vi "SO55 Settings.vi"(0 "Error In":errorcluster) -> (1 "Settings Out":T1, 2 "Error Out":errorcluster)   [LabVIEW 2012]
panel:
  in  "OK Button":bool
  in  "Settings In":T1
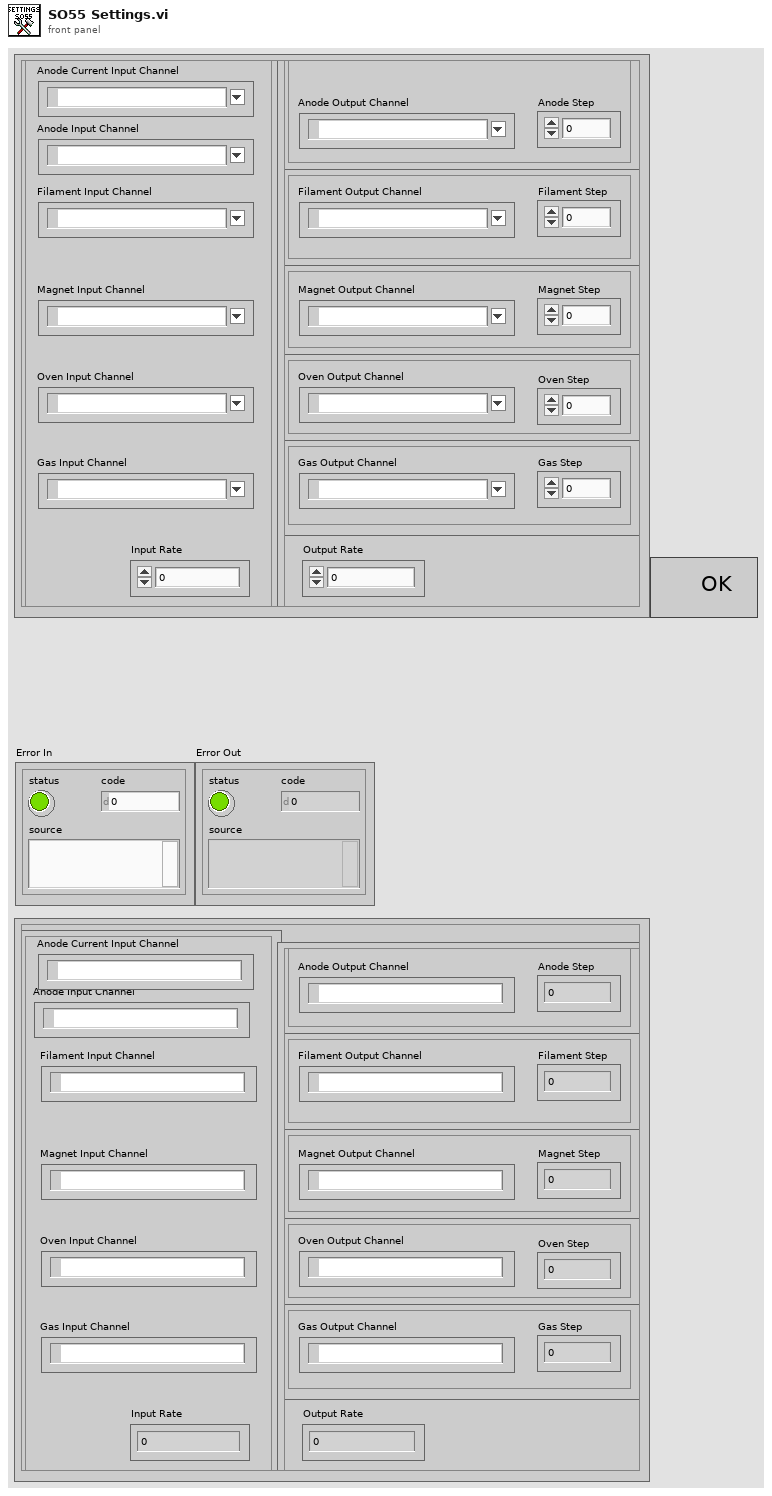
[diagram p1: front panel]
types:
  T1 = cluster{"Input":cluster{"Anode Input Channel":tag, "Filament Input Channel":tag, "Magnet Input Channel":tag, "Oven Input Channel":tag, "Gas Input Channel":tag, "Input Rate":dbl, "Anode Current Input Channel":tag}, "Output":cluster{"Anode":cluster{"Anode Output Channel":tag, "Anode Step":dbl}, "Filament":cluster{"Filament Output Channel":tag, "Filament Step":dbl}, "Magnet":cluster{"Magnet Output Channel":tag, "Magnet Step":dbl}, "Oven":cluster{"Oven Output Channel":tag, "Oven Step":dbl}, "Gas":cluster{"Gas Output Channel":tag, "Gas Step":dbl}, "Output Rate":dbl}}
  T2 = enum16{"open", "replace", "create", "open or create", "replace or create", "replace or create with confirmation"}
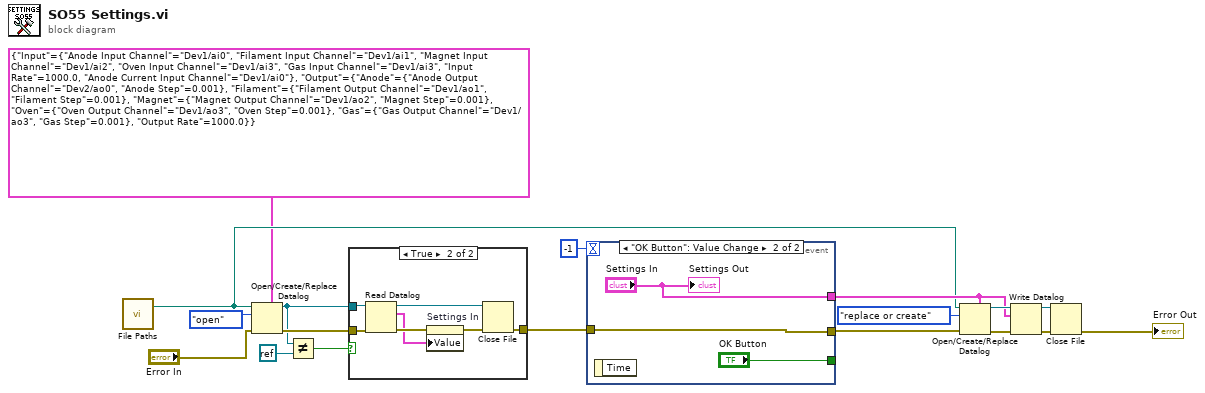
[diagram p0: block diagram]
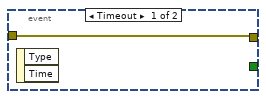
[diagram p2: hidden frame]
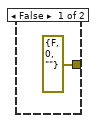
[diagram p3: hidden frame]
diagram:
  n1 = call "File Paths.vi"() -> ("SO55 Settings path"=w3:path)  [unwired: 1 out]
  n2 = Open/Create/Replace Datalog(5:T1 {"Input"={"Anode Input Channel"="Dev1/ai0", "Filament Input Channel"="Dev1/ai1", "Magnet Input Channel"="Dev1/ai2", "Oven Input Channel"="Dev1/ai3", "Gas Input Channel"="Dev1/ai3", "Input Rate"=1000.0, "Anode Current Input Channel"="Dev1/ai0"}, "Output"={"Anode"={"Anode Output Channel"="Dev2/ao0", "Anode Step"=0.001}, "Filament"={"Filament Output Channel"="Dev1/ao1", "Filament Step"=0.001}, "Magnet"={"Magnet Output Channel"="Dev1/ao2", "Magnet Step"=0.001}, "Oven"={"Oven Output Channel"="Dev1/ao3", "Oven Step"=0.001}, "Gas"={"Gas Output Channel"="Dev1/ao3", "Gas Step"=0.001}, "Output Rate"=1000.0}}, 8:"Error In", 10:T2."open" ("operation (0:open)"), 11:w3) -> (0:w16:errorcluster, 3:w15:refnum<k1>)  [unwired: 2 in, 1 out]
  n3 = Not Equal?(x=w15, y=refnum<k0> refnum) -> (x != y?=w17:bool)
  n4 = case shown="True" w17 {
    tunnel: w16 -> [_ w26]
    tunnel: w15 -> [_ w21]
    tunnel: [errorcluster {"status"=FALSE, "code"=0, "source"=""} ("error out") w22] -> w13
    frame False {
    }
    frame True {
      n5 = Read Datalog(4:w26, 7:w21) -> (0:w25:errorcluster, 2:w20:T1, 3:w23:refnum<k1>)  [unwired: 1 in]
      n6 = property on="Settings In" class="Clust (strict)"(error in=w25, "Value"=w20) -> (error out=w24:errorcluster)  [unwired: 1 in, 1 out]
      n7 = Close File(refnum=w23, error in=w24) -> (error out=w22:errorcluster)  [unwired: 1 out]
    }
  }
  n8 = event shown="[1] \"OK Button\": Value Change" {
    selector: _ -> [_ _]
    dyn-events: _ -> [_ _]
    timeout: -1 -> [_ _]
    tunnel: w13 -> [w27 w29]
    tunnel: [_ "OK Button"] -> _
    tunnel: [w27 w29] -> w11
    tunnel: [_ "Settings In"] -> w5
    event Timeout {
      n9 = event-data() -> ()  [unwired: 1 in, 2 out]
    }
    event "OK Button": Value Change {
      n10 = event-data() -> ()  [unwired: 1 in, 1 out]
      "Settings Out" <- "Settings In"
    }
  }
  n11 = Open/Create/Replace Datalog(5:w5, 8:w11, 10:T2."replace or create" ("operation (0:open)"), 11:w3) -> (0:w6:errorcluster, 3:w7:refnum<k1>)  [unwired: 2 in, 1 out]
  n12 = Write Datalog(4:w6, 6:w5, 7:w7) -> (0:w9:errorcluster, 3:w8:refnum<k1>)
  n13 = Close File(refnum=w8, error in=w9) -> (error out=→"Error Out":errorcluster)  [unwired: 1 out]
